vi "Puff_3realisation_display.vi"(2 "Actual Sampling rate (Hz)":dbl=1000.0 format="%.2f", 3 "Input Array":dbl[](array[numeric]) format="%.2f") -> ()   [LabVIEW 2010]
panel:
  in  "Case Constant\n(See Context Help)":bool
  in  "Plot3":bool
  in  "Plot2":bool
  in  "Ensample Average":cluster{dbl, dbl, dbl[]}(graph)={0.0, 0.005, array[6946 elements]}
  out "Puff Trace":cluster{dbl, dbl, dbl[]}[](graph)
  out "Puff Trace 2":cluster{dbl, dbl, dbl[]}[](graph)
  out "Puff Trace 3":cluster{dbl, dbl, dbl[]}[](graph)
  # "3 Seconds"
  # "30 seconds"
  # "0.3 seconds"
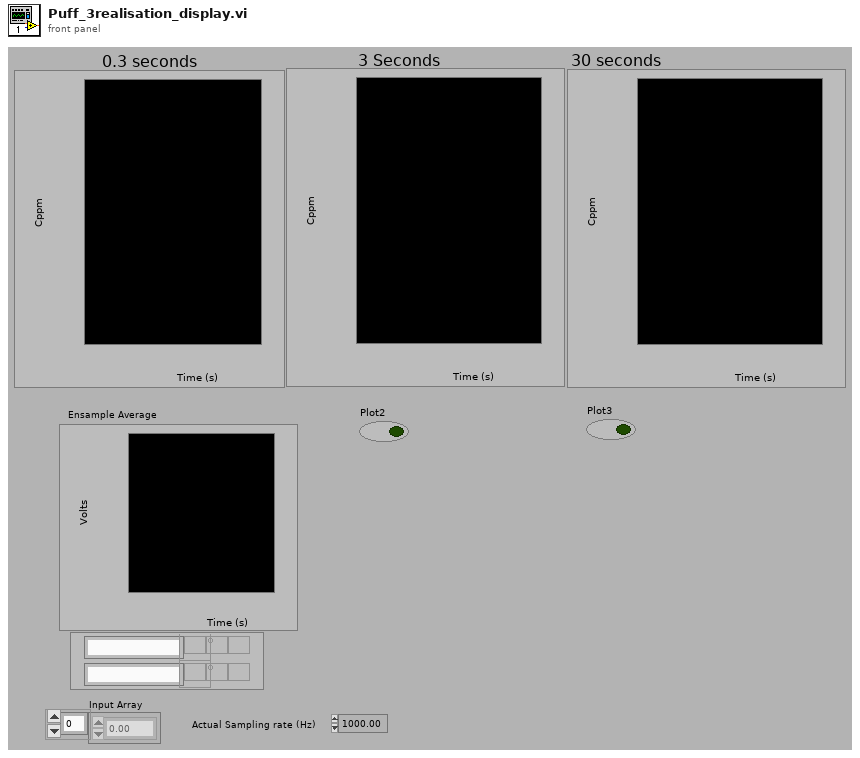
[diagram p1: front panel]
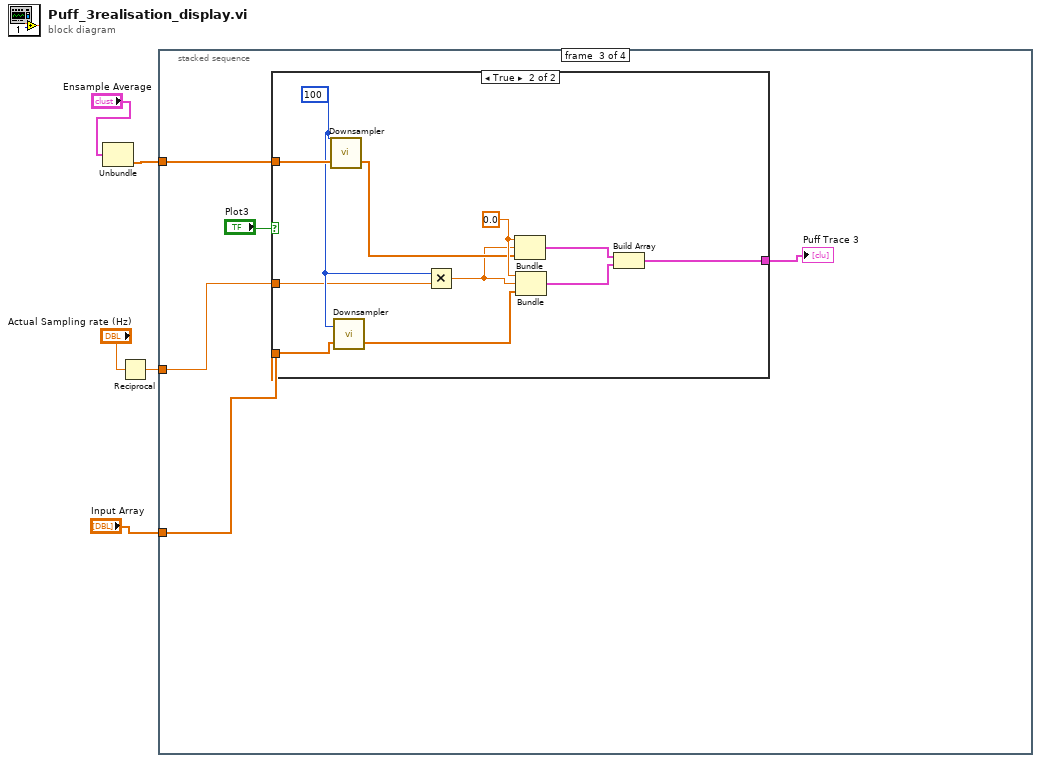
[diagram p0: block diagram]
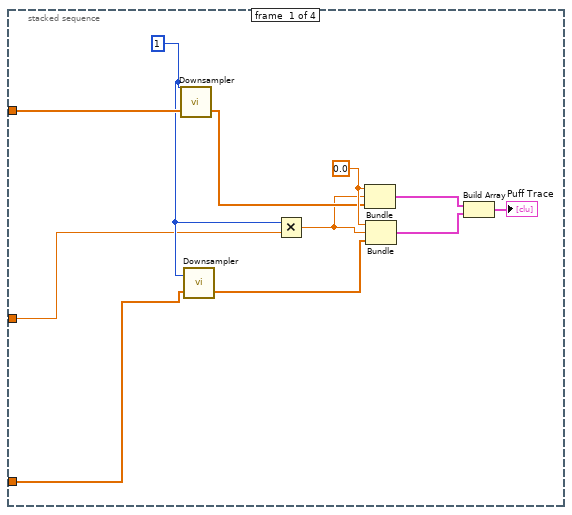
[diagram p2: hidden frame]
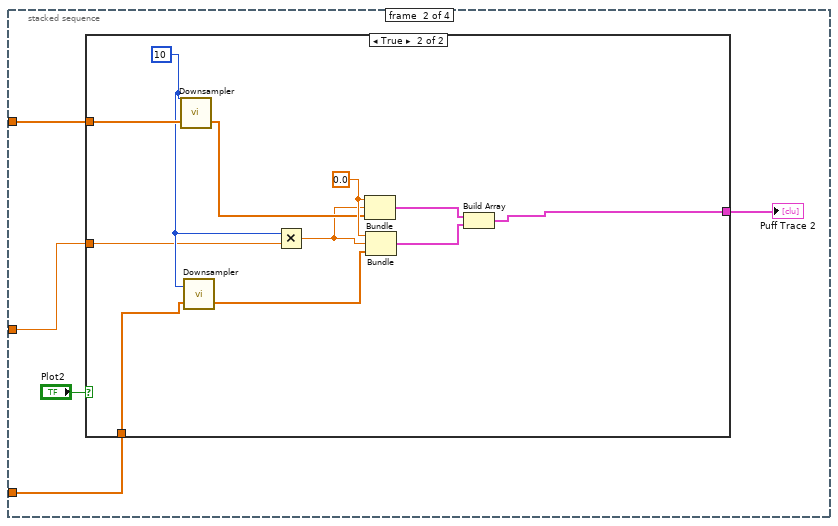
[diagram p3: hidden frame]
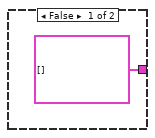
[diagram p4: hidden frame]
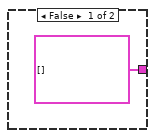
[diagram p5: hidden frame]
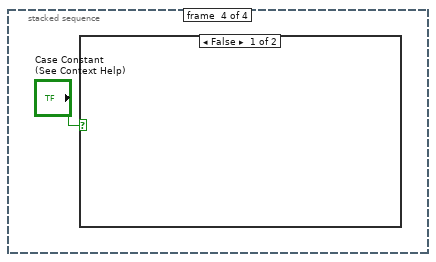
[diagram p6: hidden frame]
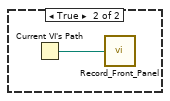
[diagram p7: hidden frame]
diagram:
  n1 = Unbundle("Ensample Average") -> (w4:dbl[])  [unwired: 2 out]
  n2 = Reciprocal(x="Actual Sampling rate (Hz)") -> (1/x=w1:dbl)
  n3 = stacked-sequence {
    tunnel: w4 -> [w16 w21 w38 _]
    tunnel: "Input Array" -> [w15 w20 w37 _]
    tunnel: w1 -> [w10 w19 w36 _]
    frame #0 {
      w11 = 1
      w14 = 0.0
      n4 = call "Downsampler.vi"("Input Array"=w16, "Averaging samples"=w11) -> ("Downsampled Array"=w12:dbl[])  [unwired: 1 out]
      n5 = call "Downsampler.vi"("Input Array"=w15, "Averaging samples"=w11) -> ("Downsampled Array"=w13:dbl[])  [unwired: 1 out]
      n6 = Multiply(x=w11, y=w10) -> (x*y=w9:dbl)
      n7 = Bundle(w14, w9, "Downsampled Array"=w12) -> (w7:cluster{dbl, dbl, "Downsampled Array":dbl[]})  [unwired: 1 in]
      n8 = Bundle(w14, w9, "Downsampled Array"=w13) -> (w8:cluster{dbl, dbl, "Downsampled Array":dbl[]})  [unwired: 1 in]
      n9 = Build Array(w7, w8) -> (→"Puff Trace":cluster{dbl, dbl, "Downsampled Array":dbl[]}[])
    }
    frame #1 {
      n10 = case shown="True" "Plot2" {
        tunnel: w21 -> [_ w33]
        tunnel: w20 -> [_ w32]
        tunnel: w19 -> [_ w27]
        tunnel: [cluster{dbl, dbl, "Downsampled Array":dbl[]}[] [] w23] -> w18
        frame False {
        }
        frame True {
          w28 = 10
          w31 = 0.0
          n11 = call "Downsampler.vi"("Input Array"=w33, "Averaging samples"=w28) -> ("Downsampled Array"=w29:dbl[])  [unwired: 1 out]
          n12 = call "Downsampler.vi"("Input Array"=w32, "Averaging samples"=w28) -> ("Downsampled Array"=w30:dbl[])  [unwired: 1 out]
          n13 = Multiply(x=w28, y=w27) -> (x*y=w26:dbl)
          n14 = Bundle(w31, w26, "Downsampled Array"=w29) -> (w24:cluster{dbl, dbl, "Downsampled Array":dbl[]})  [unwired: 1 in]
          n15 = Bundle(w31, w26, "Downsampled Array"=w30) -> (w25:cluster{dbl, dbl, "Downsampled Array":dbl[]})  [unwired: 1 in]
          n16 = Build Array(w24, w25) -> (w23:cluster{dbl, dbl, "Downsampled Array":dbl[]}[])
        }
      }
      "Puff Trace 2" <- w18
    }
    frame #2 {
      n17 = case shown="True" "Plot3" {
        tunnel: w38 -> [_ w50]
        tunnel: w37 -> [_ w49]
        tunnel: w36 -> [_ w44]
        tunnel: [cluster{dbl, dbl, "Downsampled Array":dbl[]}[] [] w40] -> w34
        frame False {
        }
        frame True {
          w45 = 100
          w48 = 0.0
          n18 = call "Downsampler.vi"("Input Array"=w50, "Averaging samples"=w45) -> ("Downsampled Array"=w46:dbl[])  [unwired: 1 out]
          n19 = call "Downsampler.vi"("Input Array"=w49, "Averaging samples"=w45) -> ("Downsampled Array"=w47:dbl[])  [unwired: 1 out]
          n20 = Multiply(x=w45, y=w44) -> (x*y=w43:dbl)
          n21 = Bundle(w48, w43, "Downsampled Array"=w46) -> (w41:cluster{dbl, dbl, "Downsampled Array":dbl[]})  [unwired: 1 in]
          n22 = Bundle(w48, w43, "Downsampled Array"=w47) -> (w42:cluster{dbl, dbl, "Downsampled Array":dbl[]})  [unwired: 1 in]
          n23 = Build Array(w41, w42) -> (w40:cluster{dbl, dbl, "Downsampled Array":dbl[]}[])
        }
      }
      "Puff Trace 3" <- w34
    }
    frame #3 {
      n24 = case shown="False" "Case Constant\n(See Context Help)" {
        frame False {
        }
        frame True {
          n25 = Current VI's Path() -> (path=w52:path)
          n26 = call "Record_Front_Panel.vi"("VI to Log"=w52) -> ()  [unwired: 1 in]
        }
      }
    }
  }
